vi "Read Amphipods.vi"(8 "error in (no error)":errorcluster, 11 "Burrow in":refnum<class "Burrow.lvclass">) -> (0 "error out":errorcluster, 2 "Amphipods":refnum<class "Amphipod.lvclass">[](array[class]), 3 "Burrow out":refnum<class "Burrow.lvclass">)   [LabVIEW 2019, in "23.lvlib" / "Burrow.lvclass"]
uses:
  Burrow.lvclass
  Amphipod/Amphipod.lvclass
  Burrow.lvclass/Burrow.ctl
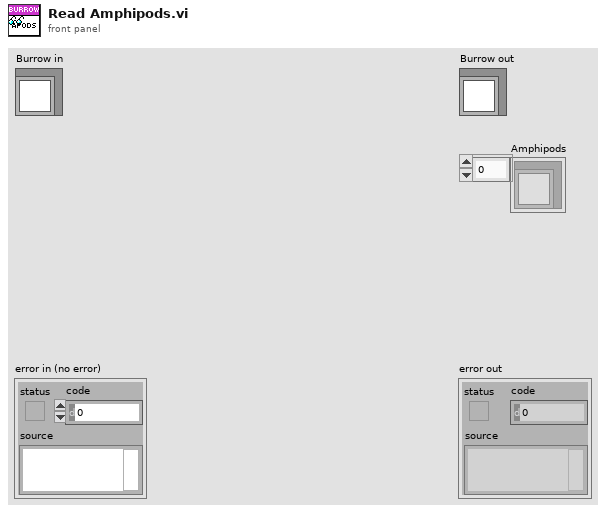
[diagram p1: front panel]
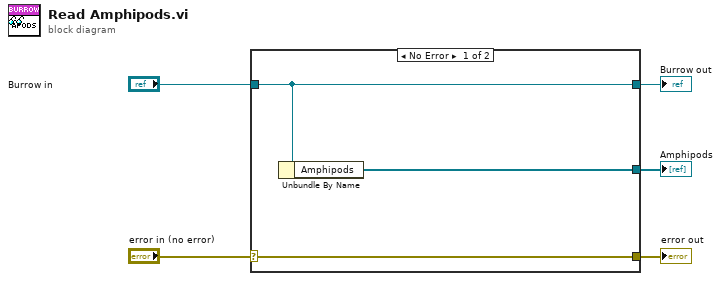
[diagram p0: block diagram]
diagram:
  n1 = case shown="No Error" "error in (no error)" {
    selector: "error in (no error)" -> [w8 w9]
    tunnel: [w8 w9] -> w4
    tunnel: [w7 w10] -> w2
    tunnel: "Burrow in" -> [w7 w10]
    tunnel: [w6 _] -> w1
    frame No Error {
      n2 = Unbundle By Name(w7) -> ("Amphipods"=w6:refnum<class "Amphipod.lvclass">[])
    }
    frame Error {
    }
  }
  "error out" <- w4
  "Burrow out" <- w2
  "Amphipods" <- w1
